vi "mbed-read Hello World.vi"() -> ()   [LabVIEW 2009]
panel:
  in  "stop":bool
  in  "Serial Port":refnum<visa-resource-name>
  out "Gauge":dbl(knob) scale=0.0..1.0
  out "Waveform Chart":dbl(graph)
  # "http://mbed.org"
  # "mbed-read Hello World!"
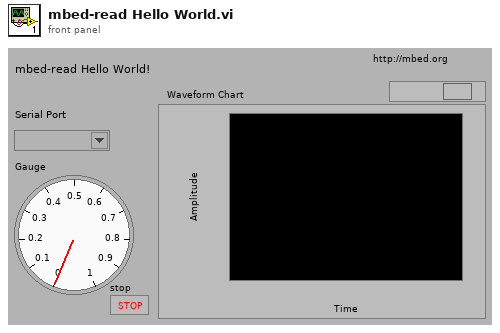
[diagram p1: front panel]
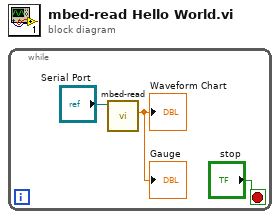
[diagram p0: block diagram]
diagram:
  n1 = while {
    stop <- "stop" stop-if-true
    n2 = call "mbed-read.vi"("Serial Port"="Serial Port") -> ("Number"=→"Waveform Chart" →"Gauge":dbl)  [unwired: 3 in, 3 out]
  }
